vi "Remove Segments From Numbers.vi"(9 "Pattern For Letter Of Letters B":string, 10 "Pattern For Number Of Letters A":string, 11 "Array":string[][](array[string])) -> (3 "Result":string)   [LabVIEW 2019, in "Day 8.lvlib"]
uses:
  Day 8.lvlib
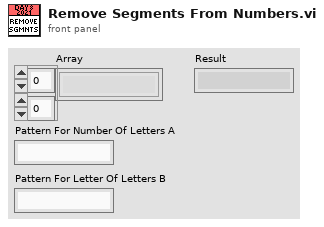
[diagram p1: front panel]
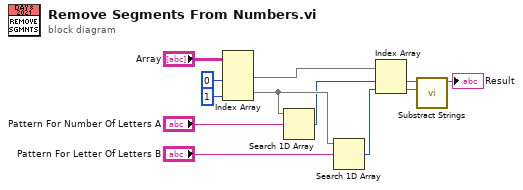
[diagram p0: block diagram]
diagram:
  n1 = Index Array(array="Array", index (col) #1=0 ("disabled index (col)"), index (col) #2=1 ("disabled index (col)")) -> (element #1=w5:string[], element #2=w7:string[])  [unwired: 2 in]
  n2 = Search 1D Array(1D array=w7, element="Pattern For Number Of Letters A") -> (index of element=w6:i32)  [unwired: 1 in]
  n3 = Search 1D Array(1D array=w7, element="Pattern For Letter Of Letters B") -> (index of element=w9:i32)  [unwired: 1 in]
  n4 = Index Array(array=w5, index #1=w6, index #2=w9) -> (element #1=w10:string, element #2=w11:string)
  n5 = call "Substract Strings.vi"("format string 2"=w11, "format string"=w10) -> ("substracted string"=→"Result":string)  [unwired: 9 in]
